vi "OG_1000_main__.vi"() -> ()   [LabVIEW 2015]
doc: "Программа мониторинга температуры ОГ-1000"
uses:
  <vilib>/NI/Modbus Library/API/Master/Modbus Master.lvclass
  <vilib>/Utility/error.llb/DialogType.ctl
panel:
  out "Связь с блоком 3":bool
  out "Связь с блоком 4":bool
  in  "Tab Control":enum32{"МНЕМОСХЕМА [K]", "R [Ом]", "НАСТРОЙКИ"}(tab)
  in  "dt 3_ch_visible":bool=TRUE
  in  "dt 2_ch_visible":bool=TRUE
  in  "dt 1_ch_visible":bool=TRUE
  out "dT3 2":dbl format="%.2f"
  out "dT2 2":dbl format="%.2f"
  out "dT1 2":dbl format="%.2f"
  in  "6_ch_visible":bool=TRUE
  in  "5_ch_visible":bool=TRUE
  in  "7_ch_visible":bool=TRUE
  in  "4_ch_visible":bool=TRUE
  in  "3_ch_visible":bool=TRUE
  in  "2_ch_visible":bool=TRUE
  in  "1_ch_visible":bool=TRUE
  out "T77":dbl format="%.2f"
  out "T66":dbl format="%.2f"
  out "T55":dbl format="%.2f"
  out "T44":dbl format="%.2f"
  out "T33":dbl format="%.2f"
  out "T22":dbl format="%.2f"
  out "T11":dbl format="%.2f"
  out "T7":dbl format="%.2f"
  out "dT3":dbl format="%.2f"
  out "T6":dbl format="%.2f"
  out "T5":dbl format="%.2f"
  out "dT2":dbl format="%.2f"
  out "T4":dbl format="%.2f"
  out "T3":dbl format="%.2f"
  out "T1":dbl format="%.2f"
  out "T2":dbl format="%.2f"
  out "dT1":dbl format="%.2f"
  out "R1":dbl format="%.2f"
  out "R2":dbl format="%.2f"
  out "R3":dbl format="%.2f"
  out "R6":dbl format="%.2f"
  out "R7":dbl format="%.2f"
  out "R5":dbl format="%.2f"
  out "R4":dbl format="%.2f"
  in  "Т min dt":dbl=4.0 min=-10.0 max=350.0 step=0.1
  in  "Т max dt":dbl=300.0 min=2.0 max=500.0 step=0.1
  in  "Autoscale dt":bool=TRUE
  in  "Порт Блока 3":u16
  in  "IP Блока 3":string
  out "Путь к файлу с коэф.":path
  in  "Пароль":string
  in  "настр. коэфф.":bool caption="Disconn"
  in  "Coeff_cl_ch5":T1 caption="T5" {"R0" format="%#_16g"; "k7" format="%#_16g"; "k6" format="%#_16g"; "k5" format="%#_16g"; "k4" format="%#_16g"; "k3" format="%#_16g"; "k2" format="%#_16g"; "k1" format="%#_16g"}
  in  "Coeff_cl_ch2":T1={"k1"=31.9101907935109921, "k2"=-399.867376562207937, "k3"=2119.32627579197288, "k4"=-5531.15447566658258, "k5"=7772.21873644739389, "k6"=-5292.23886113613844, "k7"=1613.2211984321475, "R0"=1613.2211984321475} caption="T2" {"R0" format="%#_16g"; "k7" format="%#_16g"; "k6" format="%#_16g"; "k5" format="%#_16g"; "k4" format="%#_16g"; "k3" format="%#_16g"; "k2" format="%#_16g"; "k1" format="%#_16g"}
  in  "load_coeff.":bool caption="Disconn"
  in  "save_coeff.":bool caption="Disconn"
  in  "Coeff_cl_ch4":T1 caption="T4" {"R0" format="%#_16g"; "k6" format="%#_16g"; "k5" format="%#_16g"; "k4" format="%#_16g"; "k3" format="%#_16g"; "k2" format="%#_16g"; "k1" format="%#_16g"; "k7" format="%#_16g"}
  in  "Coeff_cl_ch3":T1 caption="T3" {"R0" format="%#_16g"; "k6" format="%#_16g"; "k5" format="%#_16g"; "k4" format="%#_16g"; "k3" format="%#_16g"; "k2" format="%#_16g"; "k1" format="%#_16g"; "k7" format="%#_16g"}
  in  "Coeff_cl_ch6":T1 caption="T6" {"R0" format="%#_16g"; "k7" format="%#_16g"; "k6" format="%#_16g"; "k5" format="%#_16g"; "k4" format="%#_16g"; "k3" format="%#_16g"; "k2" format="%#_16g"; "k1" format="%#_16g"}
  in  "xScale -":bool
  in  "xScale +":bool
  out "мин.":string="1"
  in  "Добавить время":dbl(ring)=300.0 items=["10 сек."=10.0, "1 мин."=60.0, "5 мин."=300.0, "20 мин."=1200.0]
  out "часы":string="0"
  out "сек.":string="0"
  in  "stop":bool
  in  "Coeff_cl_ch1":T1 caption="T1" {"R0" format="%#_16g"; "k7" format="%#_16g"; "k6" format="%#_16g"; "k5" format="%#_16g"; "k4" format="%#_16g"; "k3" format="%#_16g"; "k2" format="%#_16g"; "k1" format="%#_16g"}
  in  "Coeff_cl_ch7":T1 caption="T7" {"R0" format="%#_16g"; "k7" format="%#_16g"; "k6" format="%#_16g"; "k5" format="%#_16g"; "k4" format="%#_16g"; "k3" format="%#_16g"; "k2" format="%#_16g"; "k1" format="%#_16g"}
  in  "GraphLookB":bool
  in  "Т min":dbl=4.0 min=-10.0 max=350.0 step=0.1
  in  "Т max":dbl=350.0 min=2.0 max=500.0 step=0.1
  in  "Autoscale":bool=TRUE
  in  "IP Блока 4":string
  in  "Порт Блока 4":u16
  out "Сутки":string
  in  "Запись в файл":bool
  out "Path":string
  out "File header exist?":bool caption="Disconn"
  in  "ADC_dyn_range":T2(ring)=enum."± 0.625 В"
  out "refnum out":refnum<file>
  out "Блок 3":refnum<class "Modbus Master.lvclass">
  out "Graphs T":dynamicdata(graph) caption="ИЗМЕРЕНИЯ ТЕМПЕРАТУРЫ, К"
  out "Блок 4":refnum<class "Modbus Master.lvclass">
  in  "Buf_size":u8=1 min=1 max=128
  in  "SPS":T3(ring)
  out "Graphs dT":dynamicdata(graph) caption="ПЕРЕПАДЫ ТЕМПЕРАТУР НА ТУРБОДЕТАНДЕРАХ, К"
  out "Расположение файла":path
  # "Блок 3"
  # "Блок 4"
  # "E51"
  # "X700"
  # "E52"
  # "D71"
  # "E53"
  # "D72"
  # "E54"
  # "X701"
  # "E61"
  # "X601"
  # "D60"
  # "C613"
  # "СБОРНИК"
  # "Шкала dТ"
  # ":"
  # ":"
  # "Шкала Т"
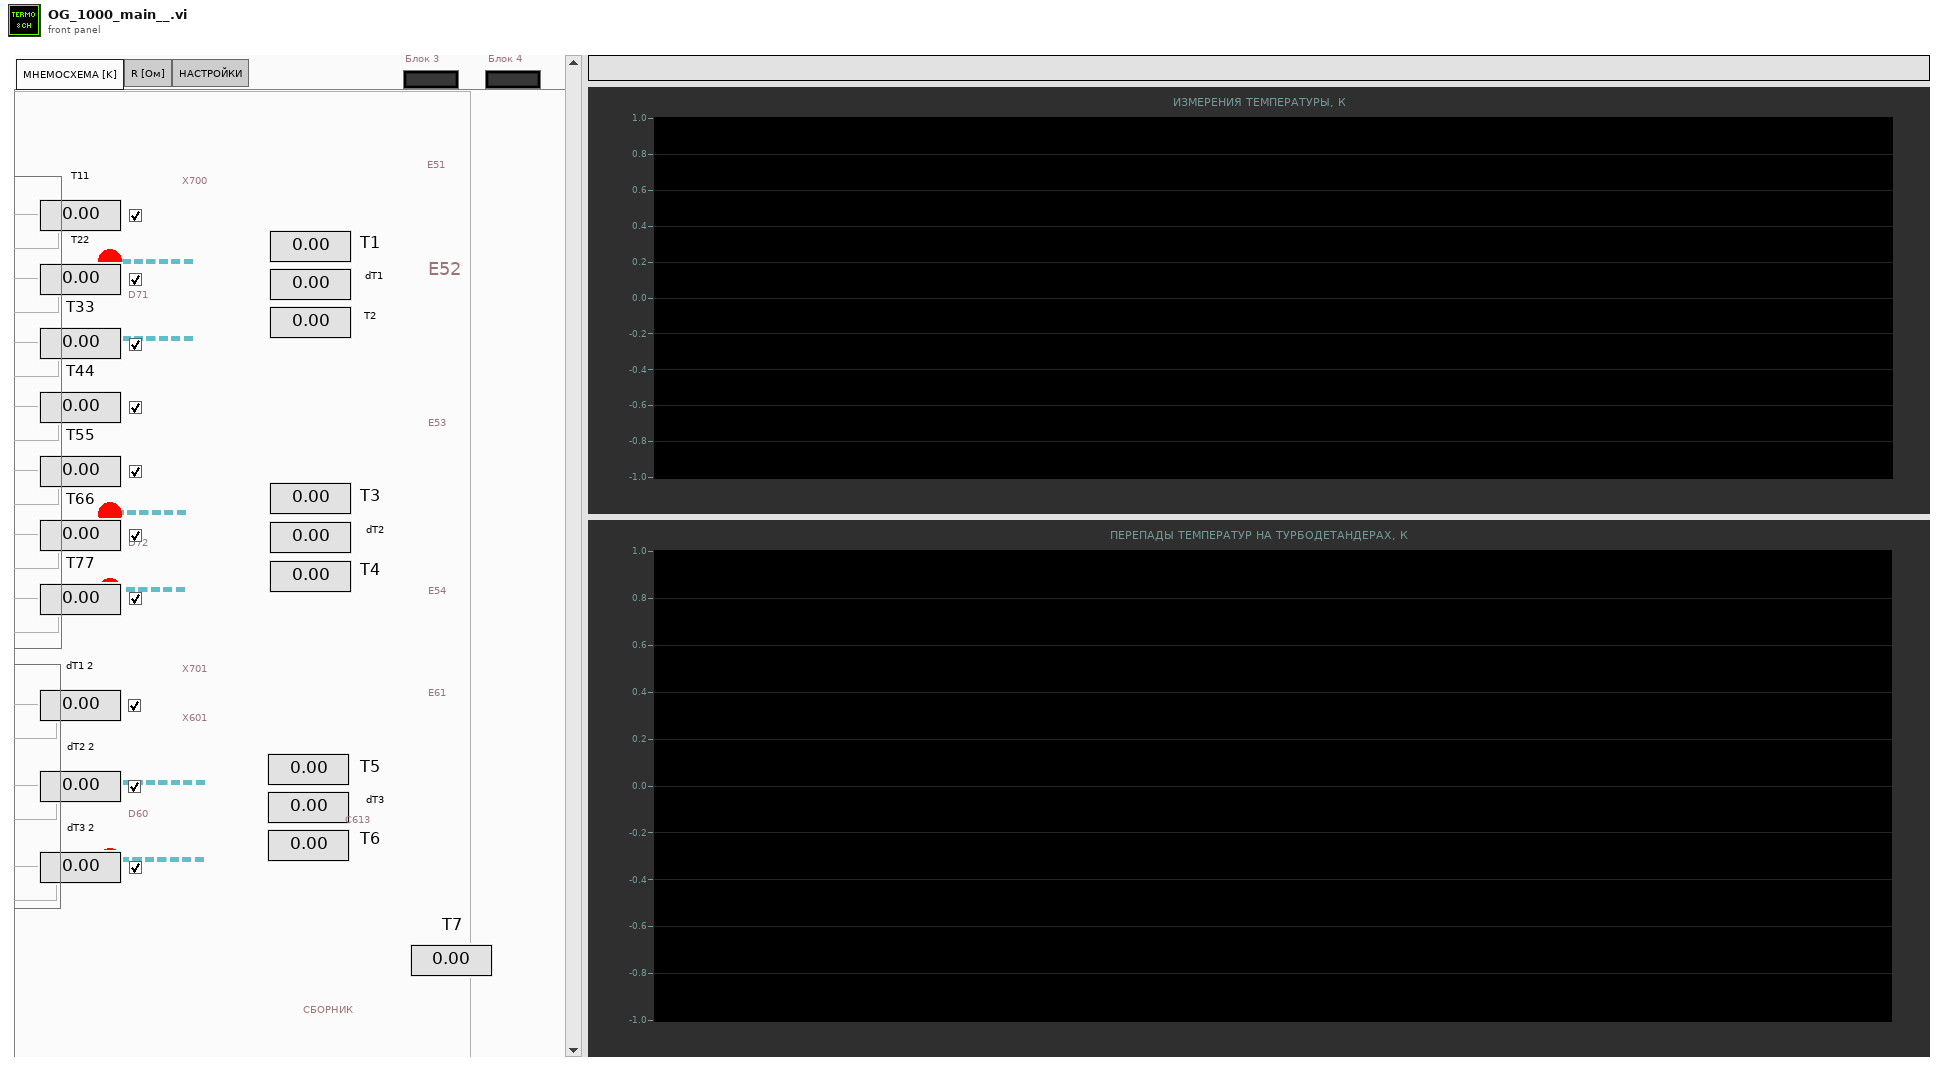
[diagram p1: front panel]
types:
  T1 = cluster{"k1":ext, "k2":ext, "k3":ext, "k4":ext, "k5":ext, "k6":ext, "k7":ext, "R0":ext}
  T2 = enum16{"± 5 В", "± 2.5 В", "± 1.25 В", "± 0.625 В", "± 312.5 мВ", "± 156.25 мВ", "± 78.125 мВ"}
  T3 = enum16{"2,5 SPS", "5 SPS", "10 SPS", "25 SPS", "50 SPS", "100 SPS", "500 SPS", "1 kSPS"}
  T4 = typedef "DialogType.ctl" = u16
  T5 = enum8{"Enabled", "Disabled", "Disabled and Grayed Out"}
  T6 = typedef "LVDateTimeRec.ctl" = cluster{"fractional second":dbl, "second":i32, "minute":i32, "hour":i32, "day of month":i32, "month":i32, "year":i32, "day of week":i32, "day of year":i32, "DST":i32}
  T7 = enum16{"open", "replace", "create", "open or create", "replace or create", "replace or create with confirmation"}
  T8 = cluster{"k1":ext, "k2":ext, "k3":ext, "k4":ext, "k5":ext, "k6":ext, "k7":ext, "R":ext}
  T9 = cluster{"T1":dbl, "T2":dbl, "T3":dbl, "T4":dbl, void, void}
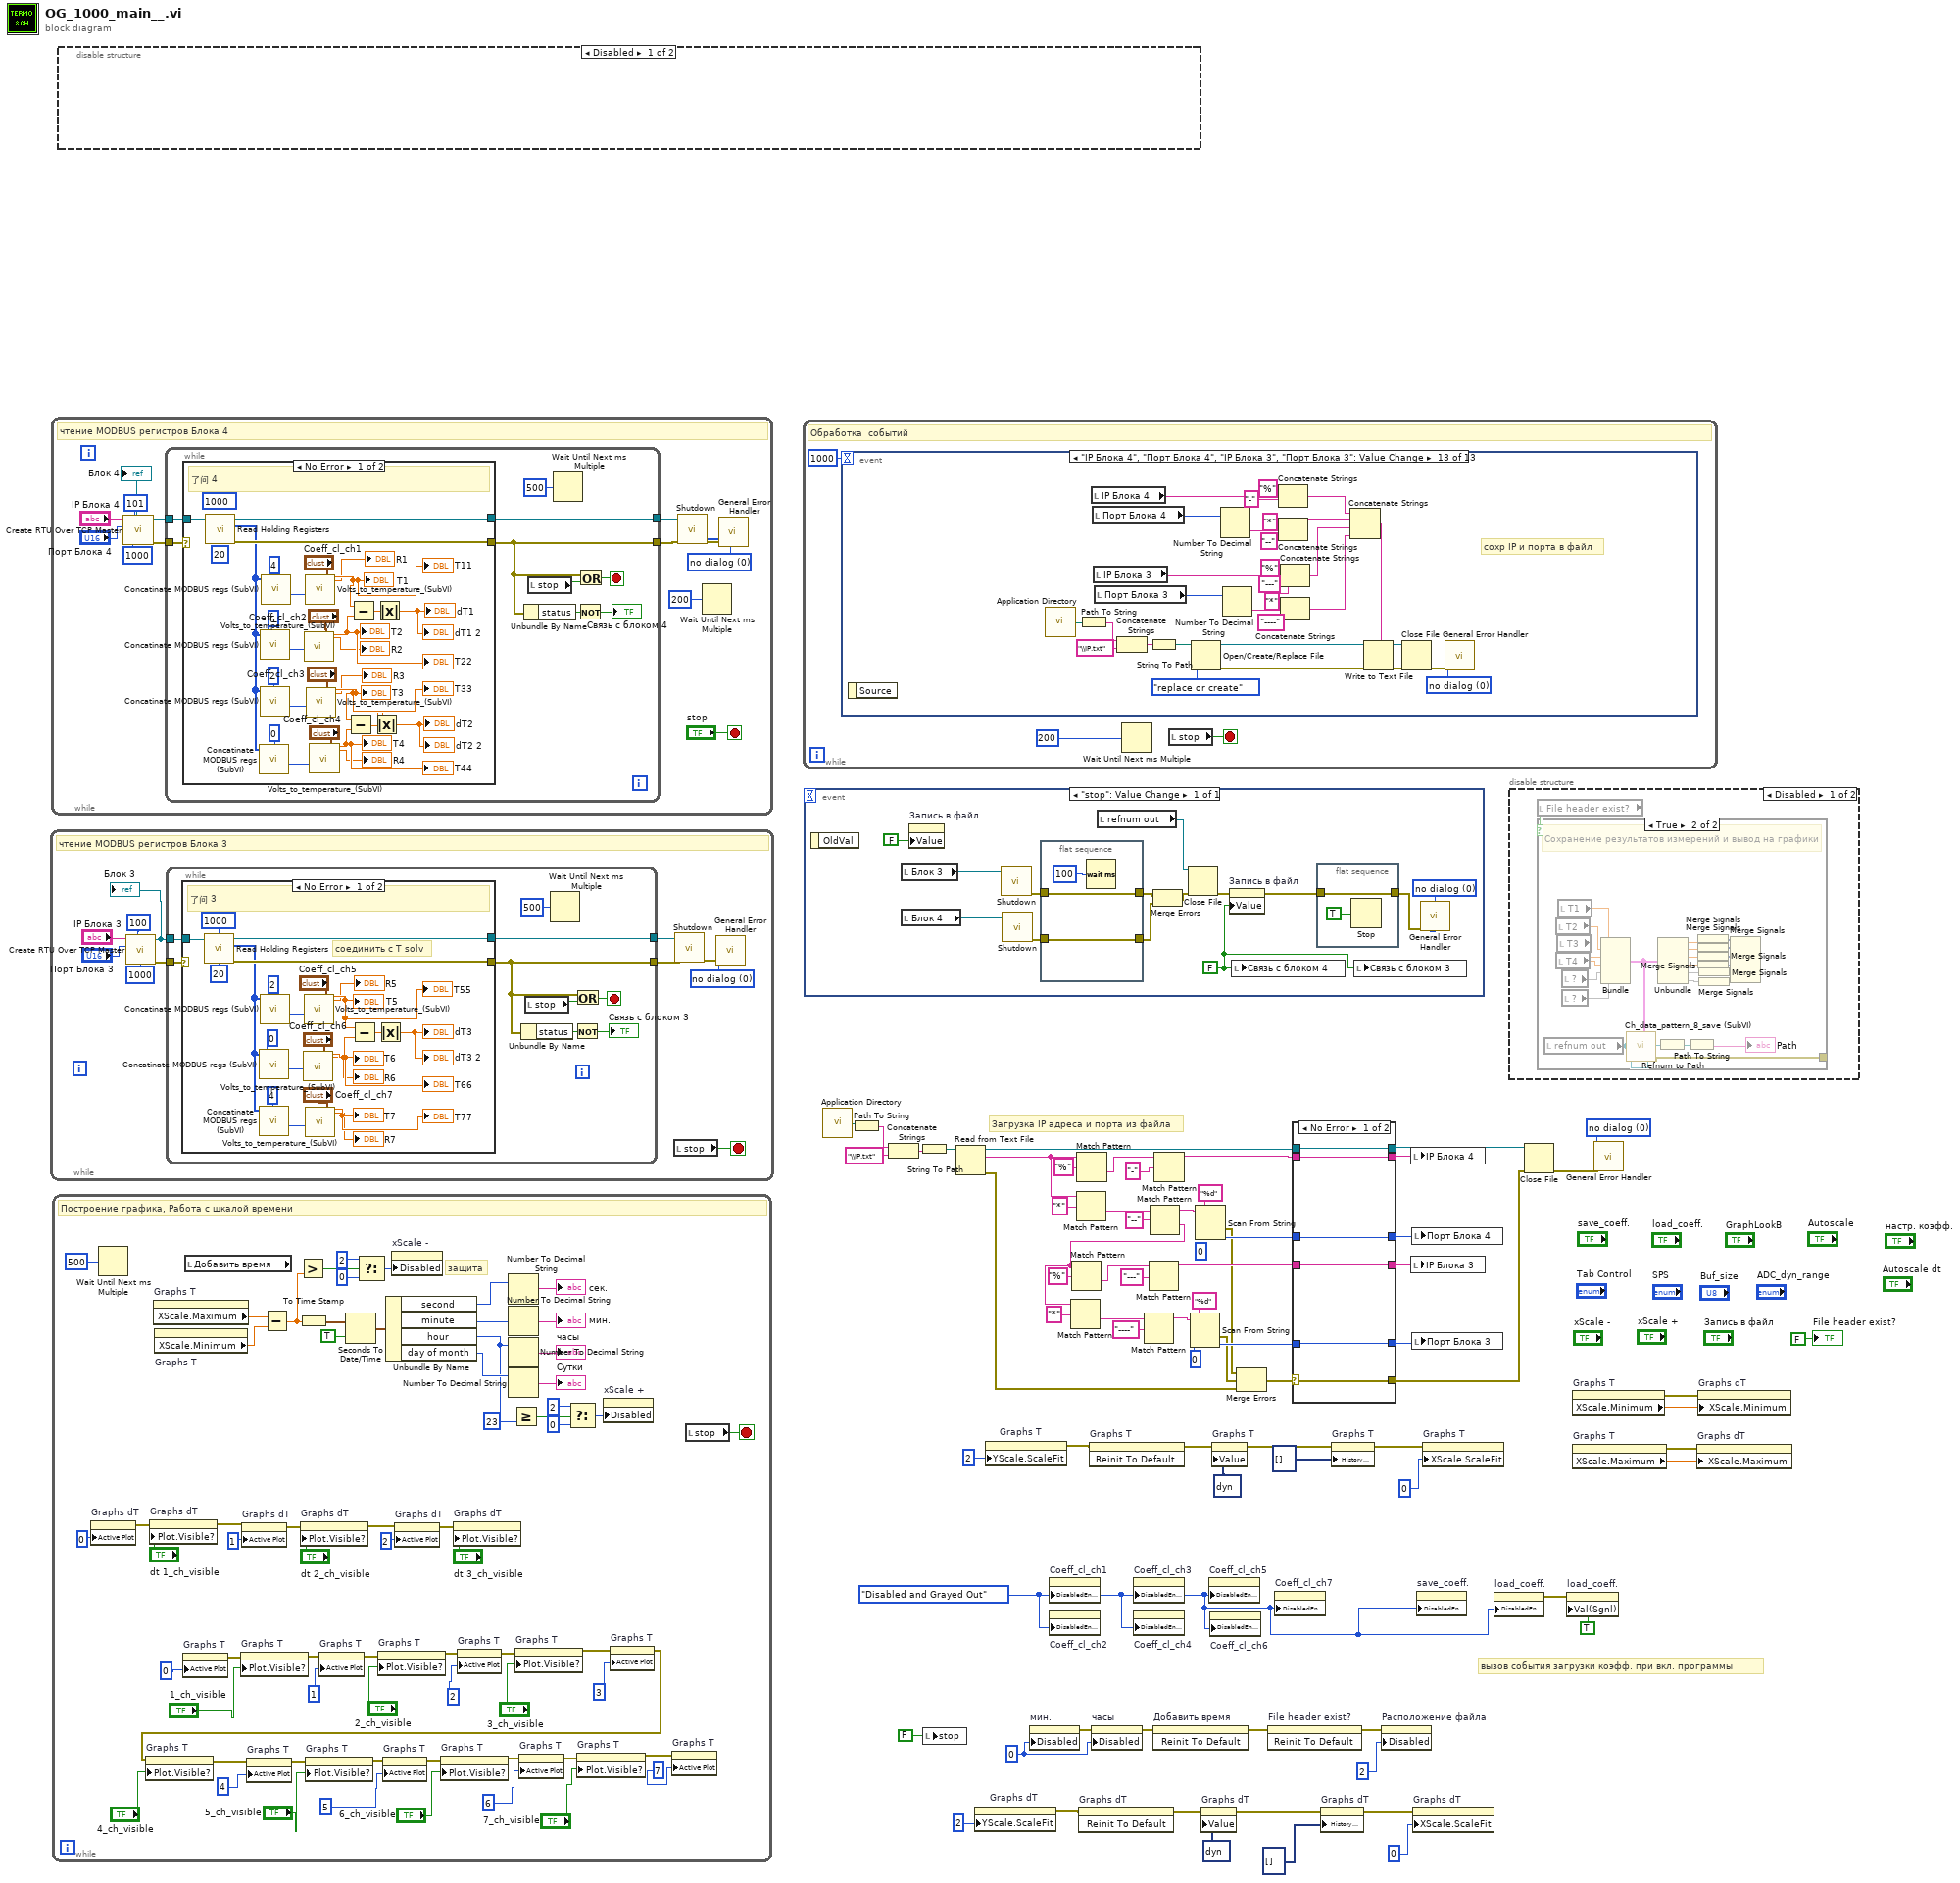
[diagram p0: block diagram]
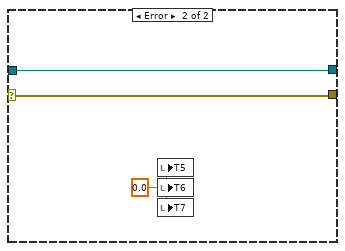
[diagram p2: hidden frame]
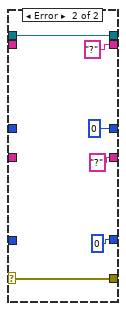
[diagram p3: hidden frame]
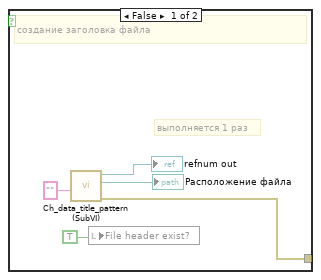
[diagram p5: hidden frame]
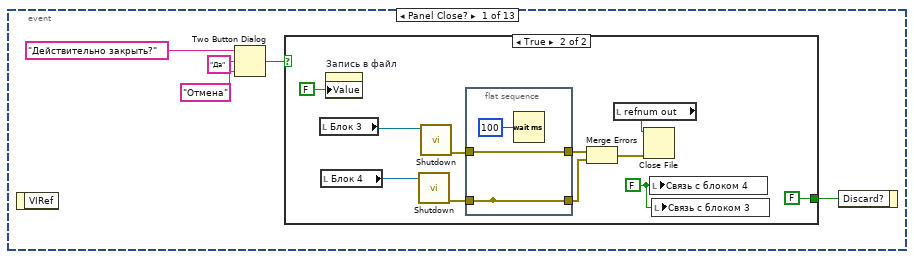
[diagram p7: hidden frame]
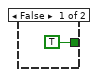
[diagram p8: hidden frame]
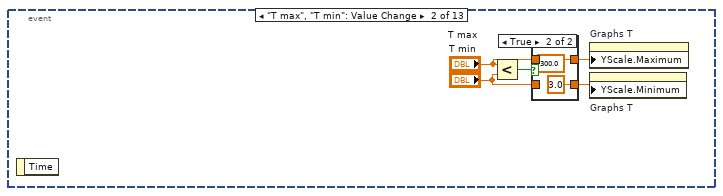
[diagram p9: hidden frame]
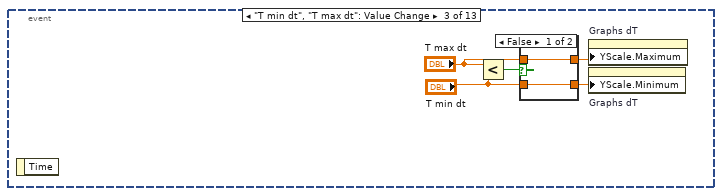
[diagram p11: hidden frame]
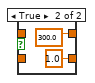
[diagram p12: hidden frame]
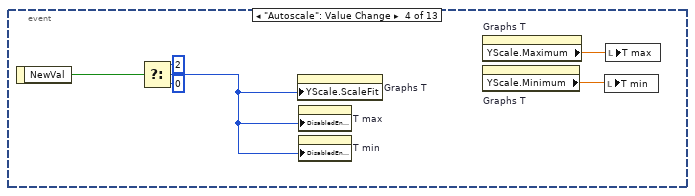
[diagram p13: hidden frame]
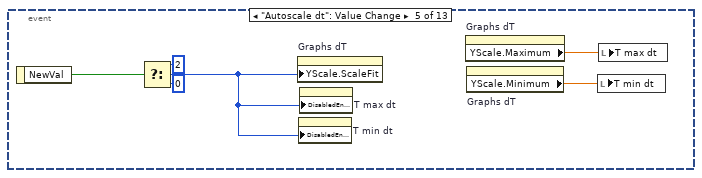
[diagram p14: hidden frame]
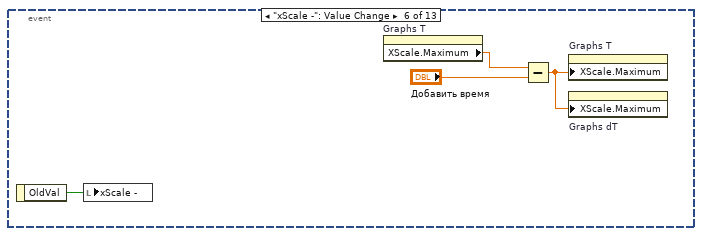
[diagram p15: hidden frame]
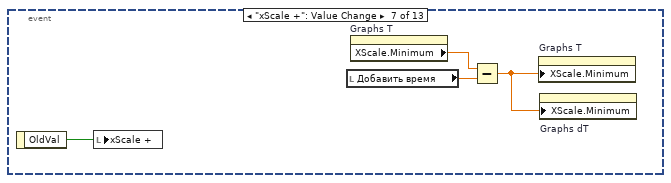
[diagram p16: hidden frame]
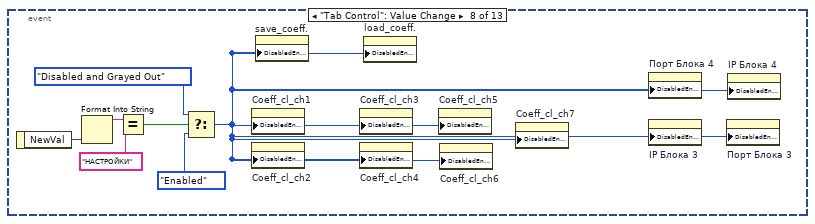
[diagram p17: hidden frame]
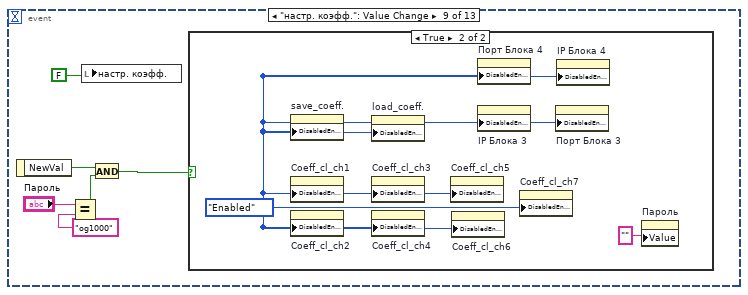
[diagram p18: hidden frame]
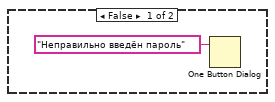
[diagram p19: hidden frame]
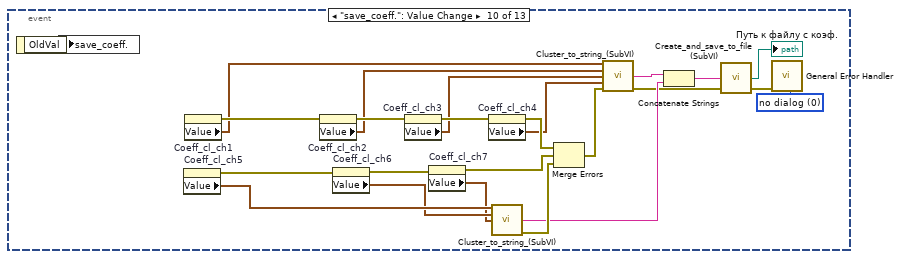
[diagram p20: hidden frame]
diagram:
  w14 = T4 0 items=["no dialog", "OK message", "continue or stop message", "OK message + warnings", "continue/stop + warnings"] ("type of dialog (OK msg:1)")
  w58 = T5."Disabled and Grayed Out" ("Disabled")
  w72 = u8 0 ("Disabled")
  # "Загрузка IP адреса и порта из файла"
  # "вызов события загрузки коэфф. при вкл. программы"
  n1 = while {
    stop <- w75 stop-if-true
    w76 = T4 0 items=["no dialog", "OK message", "continue or stop message", "OK message + warnings", "continue/stop + warnings"] ("type of dialog (OK msg:1)")
    # "чтение MODBUS регистров Блока 3"
    n2 = call "Create RTU Over TCP Master.vi"("unit ID"=u8 100 ("ID"), "connect timeout ms"=1000, "port (502)"="Порт Блока 3", "address"="IP Блока 3") -> ("error out"=w83:errorcluster, "TCP master instance"=w74:refnum<class "Modbus Master.lvclass">)  [unwired: 6 in]
    "Блок 3" <- w74
    n3 = while {
      tunnel: w74 -> [w93]
      tunnel: w83 -> [w92]
      tunnel: [w86] -> w79
      tunnel: [w91] -> w78
      stop <- w89 stop-if-true
      n4 = case shown="No Error" w92 {
        selector: w92 -> [_ w118]
        tunnel: w93 -> [w114 w119]
        tunnel: [w111 w118] -> w86
        tunnel: [w113 w119] -> w91
        frame No Error {
          # "соединить с T solv"
          # "了问 3"
          n5 = call-dynamic "Read Holding Registers.vi"("number of inputs"=u16 20, "starting address"=u16 1000, "Modbus master in"=w114) -> ("error out"=w111:errorcluster, "register values"=w107:u16[], "Modbus master out"=w113:refnum<class "Modbus Master.lvclass">)  [unwired: 6 in]
          n6 = call "Concatinate MODBUS regs (SubVI).vi"("LSB reg num"=u16 0, "registers array in"=w107) -> ("register data"=w108:i32)  [unwired: 8 in, 1 out]
          n7 = call "Concatinate MODBUS regs (SubVI).vi"("LSB reg num"=u16 4, "registers array in"=w107) -> ("register data"=w106:i32)  [unwired: 8 in, 1 out]
          n8 = call "Concatinate MODBUS regs (SubVI).vi"("LSB reg num"=u16 2, "registers array in"=w107) -> ("register data"=w110:i32)  [unwired: 8 in, 1 out]
          n9 = call "Volts_to_temperature_(SubVI).vi"("Resistance"=w108, "koeff. cluster"="Coeff_cl_ch6") -> ("T solvation"=w98:dbl, "meas_voltage"=→"R6":dbl)  [unwired: 21 in, 3 out]
          "T6" <- w98
          "T66" <- w98
          n10 = call "Volts_to_temperature_(SubVI).vi"("Resistance"=w110, "koeff. cluster"="Coeff_cl_ch5") -> ("T solvation"=w99:dbl, "meas_voltage"=→"R5":dbl)  [unwired: 21 in, 3 out]
          "T5" <- w99
          "T55" <- w99
          n11 = call "Volts_to_temperature_(SubVI).vi"("Resistance"=w106, "koeff. cluster"="Coeff_cl_ch7") -> ("T solvation"=→"T7" →"T77":dbl, "meas_voltage"=→"R7":dbl)  [unwired: 21 in, 3 out]
          n12 = Subtract(x=w99, y=w98) -> (x-y=w101:dbl)
          n13 = Absolute Value(x=w101) -> (abs(x)=→"dT3" →"dT3 2":dbl)
        }
        frame Error {
          w117 = 0.0 ("T6")
          n14 = local write "T5"(w117) -> ()
          n15 = local write "T6"(w117) -> ()
          n16 = local write "T7"(w117) -> ()
        }
      }
      n17 = Unbundle By Name(w86) -> ("status"=w88:bool)
      n18 = local read "stop"() -> (w90:bool)
      n19 = Wait Until Next ms Multiple(millisecond multiple=u32 500) -> ()  [unwired: 1 out]
      n20 = Not(x=w88) -> (.not. x?=→"Связь с блоком 3":bool)
      n21 = Or(x=w86, y=w90) -> (x .or. y?=w89:bool)
    }
    n22 = local read "stop"() -> (w75:bool)
    n23 = call-dynamic "Shutdown.vi"("error in"=w79, "Modbus master in"=w78) -> ("error out"=w80:errorcluster)  [unwired: 9 in]
    n24 = call <vilib>:"General Error Handler.vi"("type of dialog (OK msg:1)"=w76, "error in (no error)"=w80) -> ()  [unwired: 1 in, 13 out]
  }
  n25 = while {
    stop <- "stop" stop-if-true
    w120 = T4 0 items=["no dialog", "OK message", "continue or stop message", "OK message + warnings", "continue/stop + warnings"] ("type of dialog (OK msg:1)")
    # "чтение MODBUS регистров Блока 4"
    n26 = call "Create RTU Over TCP Master.vi"("unit ID"=u8 101 ("ID"), "connect timeout ms"=1000, "port (502)"="Порт Блока 4", "address"="IP Блока 4") -> ("error out"=w124:errorcluster, "TCP master instance"=w125:refnum<class "Modbus Master.lvclass">)  [unwired: 6 in]
    "Блок 4" <- w125
    n27 = while {
      tunnel: w125 -> [w140]
      tunnel: w124 -> [w139]
      tunnel: [w133] -> w123
      tunnel: [w138] -> w122
      stop <- w136 stop-if-true
      n28 = case shown="No Error" w139 {
        selector: w139 -> [_ w172]
        tunnel: w140 -> [w168 w173]
        tunnel: [w165 w172] -> w133
        tunnel: [w167 w173] -> w138
        frame No Error {
          # "了问 4"
          n29 = call-dynamic "Read Holding Registers.vi"("number of inputs"=u16 20, "starting address"=u16 1000, "Modbus master in"=w168) -> ("error out"=w165:errorcluster, "register values"=w159:u16[], "Modbus master out"=w167:refnum<class "Modbus Master.lvclass">)  [unwired: 6 in]
          n30 = call "Concatinate MODBUS regs (SubVI).vi"("LSB reg num"=u16 0, "registers array in"=w159) -> ("register data"=w154:i32)  [unwired: 8 in, 1 out]
          n31 = call "Concatinate MODBUS regs (SubVI).vi"("LSB reg num"=u16 6, "registers array in"=w159) -> ("register data"=w161:i32)  [unwired: 8 in, 1 out]
          n32 = call "Concatinate MODBUS regs (SubVI).vi"("LSB reg num"=u16 2, "registers array in"=w159) -> ("register data"=w156:i32)  [unwired: 8 in, 1 out]
          n33 = call "Concatinate MODBUS regs (SubVI).vi"("LSB reg num"=u16 4, "registers array in"=w159) -> ("register data"=w163:i32)  [unwired: 8 in, 1 out]
          n34 = call "Volts_to_temperature_(SubVI).vi"("Resistance"=w161, "koeff. cluster"="Coeff_cl_ch2") -> ("T solvation"=w148:dbl, "meas_voltage"=→"R2":dbl)  [unwired: 21 in, 3 out]
          "T2" <- w148
          "T22" <- w148
          n35 = call "Volts_to_temperature_(SubVI).vi"("Resistance"=w163, "koeff. cluster"="Coeff_cl_ch1") -> ("T solvation"=w149:dbl, "meas_voltage"=→"R1":dbl)  [unwired: 21 in, 3 out]
          "T1" <- w149
          "T11" <- w149
          n36 = call "Volts_to_temperature_(SubVI).vi"("Resistance"=w156, "koeff. cluster"="Coeff_cl_ch3") -> ("T solvation"=w147:dbl, "meas_voltage"=→"R3":dbl)  [unwired: 21 in, 3 out]
          "T3" <- w147
          "T33" <- w147
          n37 = call "Volts_to_temperature_(SubVI).vi"("Resistance"=w154, "koeff. cluster"="Coeff_cl_ch4") -> ("T solvation"=w146:dbl, "meas_voltage"=→"R4":dbl)  [unwired: 21 in, 3 out]
          "T4" <- w146
          "T44" <- w146
          n38 = Subtract(x=w147, y=w146) -> (x-y=w142:dbl)
          n39 = Subtract(x=w149, y=w148) -> (x-y=w152:dbl)
          n40 = Absolute Value(x=w142) -> (abs(x)=→"dT2" →"dT2 2":dbl)
          n41 = Absolute Value(x=w152) -> (abs(x)=→"dT1" →"dT1 2":dbl)
        }
        frame Error {
          w171 = 0.0 ("T1")
          n42 = local write "T1"(w171) -> ()
          n43 = local write "T2"(w171) -> ()
          n44 = local write "T3"(w171) -> ()
          n45 = local write "T4"(w171) -> ()
        }
      }
      n46 = Unbundle By Name(w133) -> ("status"=w135:bool)
      n47 = local read "stop"() -> (w137:bool)
      n48 = Wait Until Next ms Multiple(millisecond multiple=u32 500) -> ()  [unwired: 1 out]
      n49 = Not(x=w135) -> (.not. x?=→"Связь с блоком 4":bool)
      n50 = Or(x=w133, y=w137) -> (x .or. y?=w136:bool)
    }
    n51 = call-dynamic "Shutdown.vi"("error in"=w123, "Modbus master in"=w122) -> ("error out"=w121:errorcluster)  [unwired: 9 in]
    n52 = Wait Until Next ms Multiple(millisecond multiple=u32 200) -> ()  [unwired: 1 out]
    n53 = call <vilib>:"General Error Handler.vi"("type of dialog (OK msg:1)"=w120, "error in (no error)"=w121) -> ()  [unwired: 1 in, 13 out]
  }
  n54 = while {
    stop <- w239 stop-if-true
    # "защита"
    # "Построение графика, Работа с шкалой времени"
    n55 = property on="Graphs dT" class="WFChart (strict)"("Active Plot"=u32 0) -> (error out=w184:errorcluster)  [unwired: 2 in, 1 out]
    n56 = Wait Until Next ms Multiple(millisecond multiple=u32 500) -> ()  [unwired: 1 out]
    n57 = property on="Graphs dT" class="WFChart (strict)"(error in=w184, "Plot.Visible?"="dt 1_ch_visible") -> (error out=w178:errorcluster)  [unwired: 1 in, 1 out]
    n58 = property on="Graphs T" class="WFChart (strict)"() -> ("XScale.Maximum"=w215:dbl)  [unwired: 2 in, 2 out]
    n59 = property on="Graphs T" class="WFChart (strict)"() -> ("XScale.Minimum"=w214:dbl)  [unwired: 2 in, 2 out]
    n60 = property on="Graphs T" class="WFChart (strict)"("Active Plot"=u32 0) -> (error out=w187:errorcluster)  [unwired: 2 in, 1 out]
    n61 = local read "Добавить время"() -> (w238:dbl)
    n62 = property on="Graphs T" class="WFChart (strict)"(error in=w187, "Plot.Visible?"="1_ch_visible") -> (error out=w193:errorcluster)  [unwired: 1 in, 1 out]
    n63 = property on="Graphs dT" class="WFChart (strict)"(error in=w178, "Active Plot"=u32 1) -> (error out=w179:errorcluster)  [unwired: 1 in, 1 out]
    n64 = Subtract(x=w215, y=w214) -> (x-y=w228:dbl)
    n65 = Greater?(x=w238, y=w228) -> (0:w221:bool)
    n66 = To Time Stamp(1:w228) -> (0:w236:timestamp)
    n67 = property on="Graphs dT" class="WFChart (strict)"(error in=w179, "Plot.Visible?"="dt 2_ch_visible") -> (error out=w174:errorcluster)  [unwired: 1 in, 1 out]
    n68 = property on="Graphs T" class="WFChart (strict)"(error in=w193, "Active Plot"=u32 1) -> (error out=w190:errorcluster)  [unwired: 1 in, 1 out]
    n69 = Seconds To Date/Time(time stamp (now)=w236, to UTC (F)=TRUE) -> (date time rec=w235:T6)
    n70 = Select(t=u8 2 ("Disabled"), s=w221, f=u8 0 ("Disabled")) -> (s? t:f=w224:u8)
    n71 = property on="Graphs T" class="WFChart (strict)"(error in=w190, "Plot.Visible?"="2_ch_visible") -> (error out=w196:errorcluster)  [unwired: 1 in, 1 out]
    n72 = Unbundle By Name(w235) -> ("second"=w234:i32, "minute"=w233:i32, "hour"=w226:i32, "day of month"=w232:i32)
    n73 = property on="xScale -" class="Bool (strict)"("Disabled"=w224) -> ()  [unwired: 2 in, 2 out]
    n74 = property on="Graphs dT" class="WFChart (strict)"(error in=w174, "Active Plot"=u32 2) -> (error out=w177:errorcluster)  [unwired: 1 in, 1 out]
    n75 = property on="Graphs dT" class="WFChart (strict)"(error in=w177, "Plot.Visible?"="dt 3_ch_visible") -> ()  [unwired: 1 in, 2 out]
    n76 = property on="Graphs T" class="WFChart (strict)"(error in=w196, "Active Plot"=u32 2) -> (error out=w191:errorcluster)  [unwired: 1 in, 1 out]
    n77 = Number To Decimal String(number=w234) -> (decimal integer string=→"сек.":string)  [unwired: 1 out]
    n78 = Number To Decimal String(number=w233) -> (decimal integer string=→"мин.":string)  [unwired: 1 out]
    n79 = Number To Decimal String(number=w226) -> (decimal integer string=→"часы":string)  [unwired: 1 out]
    n80 = Number To Decimal String(number=w232) -> (decimal integer string=→"Сутки":string)  [unwired: 1 out]
    n81 = Greater Or Equal?(x=w226, y=23) -> (x >= y?=w217:bool)
    n82 = property on="Graphs T" class="WFChart (strict)"(error in=w191, "Plot.Visible?"="3_ch_visible") -> (error out=w199:errorcluster)  [unwired: 1 in, 1 out]
    n83 = Select(t=u8 2 ("Disabled"), s=w217, f=u8 0 ("Disabled")) -> (s? t:f=w220:u8)
    n84 = property on="xScale +" class="Bool (strict)"("Disabled"=w220) -> ()  [unwired: 2 in, 2 out]
    n85 = property on="Graphs T" class="WFChart (strict)"(error in=w199, "Active Plot"=u32 3) -> (error out=w185:errorcluster)  [unwired: 1 in, 1 out]
    n86 = property on="Graphs T" class="WFChart (strict)"(error in=w185, "Plot.Visible?"="4_ch_visible") -> (error out=w208:errorcluster)  [unwired: 1 in, 1 out]
    n87 = property on="Graphs T" class="WFChart (strict)"(error in=w208, "Active Plot"=u32 4) -> (error out=w206:errorcluster)  [unwired: 1 in, 1 out]
    n88 = property on="Graphs T" class="WFChart (strict)"(error in=w206, "Plot.Visible?"="5_ch_visible") -> (error out=w203:errorcluster)  [unwired: 1 in, 1 out]
    n89 = property on="Graphs T" class="WFChart (strict)"(error in=w203, "Active Plot"=u32 5) -> (error out=w205:errorcluster)  [unwired: 1 in, 1 out]
    n90 = property on="Graphs T" class="WFChart (strict)"(error in=w205, "Plot.Visible?"="6_ch_visible") -> (error out=w202:errorcluster)  [unwired: 1 in, 1 out]
    n91 = property on="Graphs T" class="WFChart (strict)"(error in=w202, "Active Plot"=u32 6) -> (error out=w204:errorcluster)  [unwired: 1 in, 1 out]
    n92 = property on="Graphs T" class="WFChart (strict)"(error in=w204, "Plot.Visible?"="7_ch_visible") -> (error out=w201:errorcluster)  [unwired: 1 in, 1 out]
    n93 = property on="Graphs T" class="WFChart (strict)"(error in=w201, "Active Plot"=u32 7) -> ()  [unwired: 1 in, 2 out]
    n94 = local read "stop"() -> (w239:bool)
  }
  n95 = disable-structure shown="Disabled" {
    frame Disabled {
    }
    frame Enabled {
    }
  }
  n96 = while {
    stop <- w241 stop-if-true
    # "Обработка  событий"
    n97 = event shown="[12] \"IP Блока 4\", \"Порт Блока 4\", \"IP Блока 3\", \"Порт Блока 3\": Value Change" {
      selector: _ -> [_ _ _ _ _ _ _ _ _ _ _ _ _]
      dyn-events: _ -> [_ _ _ _ _ _ _ _ _ _ _ _ _]
      timeout: 1000 -> [_ _ _ _ _ _ _ _ _ _ _ _ _]
      event Panel Close? {
        n98 = event-data() -> ()  [unwired: 2 out]
        n99 = Two Button Dialog(message="Действительно закрыть?", 1:"Отмена" ("T button name (\"OK\")"), 2:"Да" ("T button name (\"OK\")")) -> (T button?=w247:bool)
        n100 = case shown="True" w247 {
          tunnel: [TRUE ("Discard?") FALSE ("Discard?")] -> w243
          frame False {
          }
          frame True {
            w249 = FALSE ("Связь с блоком 4")
            n101 = local read "Блок 3"() -> (w255:refnum<class "Modbus Master.lvclass">)
            n102 = local read "Блок 4"() -> (w254:refnum<class "Modbus Master.lvclass">)
            n103 = property on="Запись в файл" class="Bool (strict)"("Value"=FALSE ("Запись в файл")) -> ()  [unwired: 2 in, 2 out]
            n104 = call-dynamic "Shutdown.vi"("Modbus master in"=w254) -> ("error out"=w253:errorcluster)  [unwired: 10 in]
            n105 = call-dynamic "Shutdown.vi"("Modbus master in"=w255) -> ("error out"=w256:errorcluster)  [unwired: 10 in]
            n106 = flat-sequence {
              tunnel: [w261] -> w252
              tunnel: w256 -> [w261]
              tunnel: w253 -> [w260]
              tunnel: [w260] -> _
              tunnel: [w260] -> w251
              frame #0 {
                n107 = Wait (ms)(milliseconds to wait=u32 100) -> ()  [unwired: 1 out]
              }
            }
            n108 = Merge Errors(w252, w251) -> (w250:errorcluster)
            n109 = local read "refnum out"() -> (w258:refnum<file>)
            n110 = Close File(refnum=w258, error in=w250) -> ()  [unwired: 2 out]
            n111 = local write "Связь с блоком 4"(w249) -> ()
            n112 = local write "Связь с блоком 3"(w249) -> ()
          }
        }
        n113 = event-data("Discard?"=w243) -> ()  [unwired: 1 in, 1 out]
      }
      event "Т max", "Т min": Value Change {
        n114 = event-data() -> ()  [unwired: 2 out]
        n115 = Less?(x="Т max", y="Т min") -> (x < y?=w267:bool)
        n116 = case shown="True" w267 {
          tunnel: [w268 300.0 ("x+1")] -> w265
          tunnel: [w269 3.0 ("x+1")] -> w266
          tunnel: "Т max" -> [w268 _]
          tunnel: "Т min" -> [w269 _]
          frame False {
          }
          frame True {
          }
        }
        n117 = property on="Graphs T" class="WFChart (strict)"("YScale.Maximum"=w265) -> ()  [unwired: 2 in, 2 out]
        n118 = property on="Graphs T" class="WFChart (strict)"("YScale.Minimum"=w266) -> ()  [unwired: 2 in, 2 out]
      }
      event "Т min dt", "Т max dt": Value Change {
        n119 = event-data() -> ()  [unwired: 2 out]
        n120 = Less?(x="Т max dt", y="Т min dt") -> (x < y?=w276:bool)
        n121 = case shown="False" w276 {
          tunnel: [w277 300.0 ("x+1")] -> w273
          tunnel: [w278 1.0 ("x+1")] -> w272
          tunnel: "Т max dt" -> [w277 _]
          tunnel: "Т min dt" -> [w278 _]
          frame False {
          }
          frame True {
          }
        }
        n122 = property on="Graphs dT" class="WFChart (strict)"("YScale.Maximum"=w273) -> ()  [unwired: 2 in, 2 out]
        n123 = property on="Graphs dT" class="WFChart (strict)"("YScale.Minimum"=w272) -> ()  [unwired: 2 in, 2 out]
      }
      event "Autoscale": Value Change {
        n124 = event-data() -> ("NewVal"=w281:bool)  [unwired: 1 out]
        n125 = Select(t=u8 2 ("Y Scale.Scale Fit"), s=w281, f=u8 0 ("Y Scale.Scale Fit")) -> (s? t:f=w284:u8)
        n126 = property on="Graphs T" class="WFChart (strict)"("YScale.ScaleFit"=w284) -> ()  [unwired: 2 in, 2 out]
        n127 = property on="Т max" class="DigNum (strict)"("DisabledEnum"=w284) -> ()  [unwired: 2 in, 2 out]
        n128 = property on="Т min" class="DigNum (strict)"("DisabledEnum"=w284) -> ()  [unwired: 2 in, 2 out]
        n129 = property on="Graphs T" class="WFChart (strict)"() -> ("YScale.Maximum"=w286:dbl)  [unwired: 2 in, 2 out]
        n130 = property on="Graphs T" class="WFChart (strict)"() -> ("YScale.Minimum"=w285:dbl)  [unwired: 2 in, 2 out]
        n131 = local write "Т min"(w285) -> ()
        n132 = local write "Т max"(w286) -> ()
      }
      event "Autoscale dt": Value Change {
        n133 = event-data() -> ("NewVal"=w290:bool)  [unwired: 1 out]
        n134 = Select(t=u8 2 ("Y Scale.Scale Fit"), s=w290, f=u8 0 ("Y Scale.Scale Fit")) -> (s? t:f=w287:u8)
        n135 = property on="Graphs dT" class="WFChart (strict)"("YScale.ScaleFit"=w287) -> ()  [unwired: 2 in, 2 out]
        n136 = property on="Т min dt" class="DigNum (strict)"("DisabledEnum"=w287) -> ()  [unwired: 2 in, 2 out]
        n137 = property on="Т max dt" class="DigNum (strict)"("DisabledEnum"=w287) -> ()  [unwired: 2 in, 2 out]
        n138 = property on="Graphs dT" class="WFChart (strict)"() -> ("YScale.Maximum"=w289:dbl)  [unwired: 2 in, 2 out]
        n139 = property on="Graphs dT" class="WFChart (strict)"() -> ("YScale.Minimum"=w288:dbl)  [unwired: 2 in, 2 out]
        n140 = local write "Т min dt"(w288) -> ()
        n141 = local write "Т max dt"(w289) -> ()
      }
      event "xScale -": Value Change {
        n142 = event-data() -> ("OldVal"=w296:bool)  [unwired: 1 out]
        n143 = local write "xScale -"(w296) -> ()
        n144 = property on="Graphs T" class="WFChart (strict)"() -> ("XScale.Maximum"=w294:dbl)  [unwired: 2 in, 2 out]
        n145 = Subtract(x=w294, y="Добавить время") -> (x-y=w293:dbl)
        n146 = property on="Graphs T" class="WFChart (strict)"("XScale.Maximum"=w293) -> ()  [unwired: 2 in, 2 out]
        n147 = property on="Graphs dT" class="WFChart (strict)"("XScale.Maximum"=w293) -> ()  [unwired: 2 in, 2 out]
      }
      event "xScale +": Value Change {
        n148 = event-data() -> ("OldVal"=w300:bool)  [unwired: 1 out]
        n149 = local write "xScale +"(w300) -> ()
        n150 = local read "Добавить время"() -> (w299:dbl)
        n151 = property on="Graphs T" class="WFChart (strict)"() -> ("XScale.Minimum"=w298:dbl)  [unwired: 2 in, 2 out]
        n152 = Subtract(x=w298, y=w299) -> (x-y=w297:dbl)
        n153 = property on="Graphs T" class="WFChart (strict)"("XScale.Minimum"=w297) -> ()  [unwired: 2 in, 2 out]
        n154 = property on="Graphs dT" class="WFChart (strict)"("XScale.Minimum"=w297) -> ()  [unwired: 2 in, 2 out]
      }
      event "Tab Control": Value Change {
        n155 = event-data() -> ("NewVal"=w307:enum32{"МНЕМОСХЕМА [K]", "R [Ом]", "НАСТРОЙКИ"})  [unwired: 1 out]
        n156 = Format Into String(w307) -> (resulting string=w306:string)  [unwired: 3 in, 1 out]
        n157 = Equal?(x=w306, y="НАСТРОЙКИ") -> (x = y?=w304:bool)
        n158 = Select(t=T5."Disabled and Grayed Out" ("Disabled"), s=w304, f=T5."Enabled" ("Disabled")) -> (s? t:f=w301:T5)
        n159 = property on="Coeff_cl_ch1" class="Clust (strict)"("DisabledEnum"=w301) -> ()  [unwired: 2 in, 2 out]
        n160 = property on="Coeff_cl_ch2" class="Clust (strict)"("DisabledEnum"=w301) -> ()  [unwired: 2 in, 2 out]
        n161 = property on="save_coeff." class="Bool (strict)"("DisabledEnum"=w301) -> ()  [unwired: 2 in, 2 out]
        n162 = property on="Coeff_cl_ch3" class="Clust (strict)"("DisabledEnum"=w301) -> ()  [unwired: 2 in, 2 out]
        n163 = property on="Coeff_cl_ch4" class="Clust (strict)"("DisabledEnum"=w301) -> ()  [unwired: 2 in, 2 out]
        n164 = property on="load_coeff." class="Bool (strict)"("DisabledEnum"=w301) -> ()  [unwired: 2 in, 2 out]
        n165 = property on="Coeff_cl_ch5" class="Clust (strict)"("DisabledEnum"=w301) -> ()  [unwired: 2 in, 2 out]
        n166 = property on="Coeff_cl_ch6" class="Clust (strict)"("DisabledEnum"=w301) -> ()  [unwired: 2 in, 2 out]
        n167 = property on="Coeff_cl_ch7" class="Clust (strict)"("DisabledEnum"=w301) -> ()  [unwired: 2 in, 2 out]
        n168 = property on="Порт Блока 4" class="DigNum (strict)"("DisabledEnum"=w301) -> ()  [unwired: 2 in, 2 out]
        n169 = property on="IP Блока 3" class="Str"("DisabledEnum"=w301) -> ()  [unwired: 2 in, 2 out]
        n170 = property on="Порт Блока 3" class="DigNum (strict)"("DisabledEnum"=w301) -> ()  [unwired: 2 in, 2 out]
        n171 = property on="IP Блока 4" class="Str"("DisabledEnum"=w301) -> ()  [unwired: 2 in, 2 out]
      }
      event "настр. коэфф.": Value Change {
        n172 = event-data() -> ("NewVal"=w313:bool)  [unwired: 1 out]
        n173 = Equal?(x="Пароль", y="og1000") -> (x = y?=w310:bool)
        n174 = local write "настр. коэфф."(FALSE ("насстр. коэфф.")) -> ()
        n175 = And(x=w313, y=w310) -> (x .and. y?=w309:bool)
        n176 = case shown="True" w309 {
          frame False {
            n177 = One Button Dialog(message="Неправильно введён пароль") -> ()  [unwired: 1 in, 1 out]
          }
          frame True {
            w315 = T5."Enabled" ("Disabled")
            n178 = property on="save_coeff." class="Bool (strict)"("DisabledEnum"=w315) -> ()  [unwired: 2 in, 2 out]
            n179 = property on="Coeff_cl_ch1" class="Clust (strict)"("DisabledEnum"=w315) -> ()  [unwired: 2 in, 2 out]
            n180 = property on="Coeff_cl_ch2" class="Clust (strict)"("DisabledEnum"=w315) -> ()  [unwired: 2 in, 2 out]
            n181 = property on="load_coeff." class="Bool (strict)"("DisabledEnum"=w315) -> ()  [unwired: 2 in, 2 out]
            n182 = property on="Coeff_cl_ch3" class="Clust (strict)"("DisabledEnum"=w315) -> ()  [unwired: 2 in, 2 out]
            n183 = property on="Coeff_cl_ch4" class="Clust (strict)"("DisabledEnum"=w315) -> ()  [unwired: 2 in, 2 out]
            n184 = property on="Coeff_cl_ch5" class="Clust (strict)"("DisabledEnum"=w315) -> ()  [unwired: 2 in, 2 out]
            n185 = property on="Coeff_cl_ch6" class="Clust (strict)"("DisabledEnum"=w315) -> ()  [unwired: 2 in, 2 out]
            n186 = property on="Порт Блока 4" class="DigNum (strict)"("DisabledEnum"=w315) -> ()  [unwired: 2 in, 2 out]
            n187 = property on="IP Блока 3" class="Str"("DisabledEnum"=w315) -> ()  [unwired: 2 in, 2 out]
            n188 = property on="Coeff_cl_ch7" class="Clust (strict)"("DisabledEnum"=w315) -> ()  [unwired: 2 in, 2 out]
            n189 = property on="Порт Блока 3" class="DigNum (strict)"("DisabledEnum"=w315) -> ()  [unwired: 2 in, 2 out]
            n190 = property on="IP Блока 4" class="Str"("DisabledEnum"=w315) -> ()  [unwired: 2 in, 2 out]
            n191 = property on="Пароль" class="Str"("Value"="" ("Пароль")) -> ()  [unwired: 2 in, 2 out]
          }
        }
      }
      event "save_coeff.": Value Change {
        w318 = T4 0 items=["no dialog", "OK message", "continue or stop message", "OK message + warnings", "continue/stop + warnings"] ("type of dialog (OK msg:1)")
        n192 = event-data() -> ("OldVal"=w340:bool)  [unwired: 1 out]
        n193 = local write "save_coeff."(w340) -> ()
        n194 = property on="Coeff_cl_ch5" class="Clust (strict)"() -> (error out=w336:errorcluster, "Value"=w327:T1)  [unwired: 2 in, 1 out]
        n195 = property on="Coeff_cl_ch1" class="Clust (strict)"() -> (error out=w339:errorcluster, "Value"=w331:T1)  [unwired: 2 in, 1 out]
        n196 = property on="Coeff_cl_ch2" class="Clust (strict)"(error in=w339) -> (error out=w338:errorcluster, "Value"=w330:T1)  [unwired: 1 in, 1 out]
        n197 = property on="Coeff_cl_ch6" class="Clust (strict)"(error in=w336) -> (error out=w335:errorcluster, "Value"=w326:T1)  [unwired: 1 in, 1 out]
        n198 = property on="Coeff_cl_ch3" class="Clust (strict)"(error in=w338) -> (error out=w337:errorcluster, "Value"=w329:T1)  [unwired: 1 in, 1 out]
        n199 = property on="Coeff_cl_ch7" class="Clust (strict)"(error in=w335) -> (error out=w332:errorcluster, "Value"=w325:T1)  [unwired: 1 in, 1 out]
        n200 = property on="Coeff_cl_ch4" class="Clust (strict)"(error in=w337) -> (error out=w333:errorcluster, "Value"=w328:T1)  [unwired: 1 in, 1 out]
        n201 = call "Cluster_to_string_(SubVI).vi"("input cluster 1"=w327, "input cluster 2"=w326, "input cluster 3"=w325) -> ("string of coefficients"=w323:string, "error out"=w324:errorcluster)  [unwired: 11 in]
        n202 = Merge Errors(w333, w332, w324) -> (w334:errorcluster)
        n203 = call "Cluster_to_string_(SubVI).vi"("input cluster 1"=w331, "input cluster 2"=w330, "input cluster 3"=w329, "input cluster 4"=w328, "error in"=w334) -> ("string of coefficients"=w322:string, "error out"=w320:errorcluster)  [unwired: 9 in]
        n204 = Concatenate Strings(w322, w323) -> (w321:string)
        n205 = call "Create_and_save_to_file (SubVI).vi"("input string"=w321, "error in"=w320) -> ("Текущее расположение файла"=→"Путь к файлу с коэф.":path, "error out"=w319:errorcluster)  [unwired: 4 in]
        n206 = call <vilib>:"General Error Handler.vi"("type of dialog (OK msg:1)"=w318, "error in (no error)"=w319) -> ()  [unwired: 9 in, 5 out]
      }
      event "load_coeff.": Value Change {
        w343 = T4 0 items=["no dialog", "OK message", "continue or stop message", "OK message + warnings", "continue/stop + warnings"] ("type of dialog (OK msg:1)")
        n207 = event-data() -> ("OldVal"=w345:bool)  [unwired: 1 out]
        n208 = disable-structure shown="Enabled" {
          disable-tunnel: [w348 w351] -> w342
          disable-tunnel: [w347 w352] -> w344
          frame Disabled {
            n209 = Read from Text File(prompt (Open existing file)="Укажите  файл") -> (text=w347:string, cancelled=w349:bool, error out=w348:errorcluster)  [unwired: 3 in, 1 out]
          }
          frame Enabled {
            n210 = call <vilib>:"Application Directory.vi"() -> ("Application Directory"=w356:path)
            n211 = Path To String(path=w356) -> (string=w355:string)
            n212 = Concatenate Strings(w355, "\\Настройки.txt" ("prompt (Open existing file)")) -> (w354:string)
            n213 = String To Path(string=w354) -> (path=w350:path)
            n214 = local write "Путь к файлу с коэф."(w350) -> ()
            n215 = Read from Text File(file (use dialog)=w350) -> (text=w352:string, error out=w351:errorcluster)  [unwired: 3 in, 2 out]
          }
        }
        n216 = local write "load_coeff."(w345) -> ()
        n217 = case shown="No Error" w342 {
          selector: w342 -> [w360 w386]
          tunnel: w344 -> [w385 _]
          tunnel: [w357 w386] -> w341
          frame No Error {
            n218 = call "String_to_num (SubVI).vi"("String in"=w385, "error in"=w360) -> ("Rest of string OUT"=w382:string, "error out"=w383:errorcluster, "output cluster \nof coefficients"=w384:T8)  [unwired: 5 in]
            n219 = property on="Coeff_cl_ch1" class="Clust (strict)"(error in=w383, "Value"=w384) -> (error out=w381:errorcluster)  [unwired: 1 in, 1 out]
            n220 = call "String_to_num (SubVI).vi"("String in"=w382, "error in"=w381) -> ("Rest of string OUT"=w365:string, "error out"=w380:errorcluster, "output cluster \nof coefficients"=w379:T8)  [unwired: 5 in]
            n221 = property on="Coeff_cl_ch2" class="Clust (strict)"(error in=w380, "Value"=w379) -> (error out=w378:errorcluster)  [unwired: 1 in, 1 out]
            n222 = call "String_to_num (SubVI).vi"("String in"=w365, "error in"=w378) -> ("Rest of string OUT"=w366:string, "error out"=w377:errorcluster, "output cluster \nof coefficients"=w364:T8)  [unwired: 5 in]
            n223 = property on="Coeff_cl_ch3" class="Clust (strict)"(error in=w377, "Value"=w364) -> (error out=w376:errorcluster)  [unwired: 1 in, 1 out]
            n224 = call "String_to_num (SubVI).vi"("String in"=w366, "error in"=w376) -> ("Rest of string OUT"=w359:string, "error out"=w375:errorcluster, "output cluster \nof coefficients"=w363:T8)  [unwired: 5 in]
            n225 = property on="Coeff_cl_ch4" class="Clust (strict)"(error in=w375, "Value"=w363) -> (error out=w358:errorcluster)  [unwired: 1 in, 1 out]
            n226 = call "String_to_num (SubVI).vi"("String in"=w359, "error in"=w358) -> ("Rest of string OUT"=w367:string, "error out"=w374:errorcluster, "output cluster \nof coefficients"=w362:T8)  [unwired: 5 in]
            n227 = property on="Coeff_cl_ch5" class="Clust (strict)"(error in=w374, "Value"=w362) -> (error out=w373:errorcluster)  [unwired: 1 in, 1 out]
            n228 = call "String_to_num (SubVI).vi"("String in"=w367, "error in"=w373) -> ("Rest of string OUT"=w368:string, "error out"=w372:errorcluster, "output cluster \nof coefficients"=w361:T8)  [unwired: 5 in]
            n229 = property on="Coeff_cl_ch6" class="Clust (strict)"(error in=w372, "Value"=w361) -> (error out=w371:errorcluster)  [unwired: 1 in, 1 out]
            n230 = call "String_to_num (SubVI).vi"("String in"=w368, "error in"=w371) -> ("error out"=w370:errorcluster, "output cluster \nof coefficients"=w369:T8)  [unwired: 5 in, 1 out]
            n231 = property on="Coeff_cl_ch7" class="Clust (strict)"(error in=w370, "Value"=w369) -> (error out=w357:errorcluster)  [unwired: 1 in, 1 out]
          }
          frame Error {
            w387 = T1 {"k1"=0.0, "k2"=0.0, "k3"=0.0, "k4"=0.0, "k5"=0.0, "k6"=0.0, "k7"=0.0, "R0"=0.0} ("Coeff_cl_ch1")
            n232 = property on="Coeff_cl_ch1" class="Clust (strict)"("Value"=w387) -> ()  [unwired: 2 in, 2 out]
            n233 = property on="Coeff_cl_ch2" class="Clust (strict)"("Value"=w387) -> ()  [unwired: 2 in, 2 out]
            n234 = property on="Coeff_cl_ch3" class="Clust (strict)"("Value"=w387) -> ()  [unwired: 2 in, 2 out]
            n235 = property on="Coeff_cl_ch4" class="Clust (strict)"("Value"=w387) -> ()  [unwired: 2 in, 2 out]
            n236 = property on="Coeff_cl_ch5" class="Clust (strict)"("Value"=w387) -> ()  [unwired: 2 in, 2 out]
            n237 = property on="Coeff_cl_ch6" class="Clust (strict)"("Value"=w387) -> ()  [unwired: 2 in, 2 out]
            n238 = String To Path(string="Ошибка загрузки файла Настройки.txt") -> (path=w389:path)
            n239 = property on="Coeff_cl_ch7" class="Clust (strict)"("Value"=w387) -> ()  [unwired: 2 in, 2 out]
            n240 = local write "Путь к файлу с коэф."(w389) -> ()
          }
        }
        n241 = call <vilib>:"General Error Handler.vi"("type of dialog (OK msg:1)"=w343, "error in (no error)"=w341) -> ()  [unwired: 9 in, 5 out]
      }
      event Timeout {
        n242 = event-data() -> ()  [unwired: 2 out]
        n243 = local read "T1"() -> (w411:dbl)
        n244 = local read "T2"() -> (w410:dbl)
        n245 = local read "T3"() -> (w409:dbl)
        n246 = local read "T4"() -> (w406:dbl)
        n247 = local read "T5"() -> (w407:dbl)
        n248 = local read "T6"() -> (w408:dbl)
        n249 = local read "T7"() -> (w405:dbl)
        n250 = Merge Signals(w411) -> (w404:dynamicdata)
        n251 = Merge Signals(w410) -> (w403:dynamicdata)
        n252 = Merge Signals(w409) -> (w402:dynamicdata)
        n253 = Merge Signals(w406) -> (w401:dynamicdata)
        n254 = Merge Signals(w407) -> (w400:dynamicdata)
        n255 = Merge Signals(w408) -> (w399:dynamicdata)
        n256 = Merge Signals(w405) -> (w398:dynamicdata)
        n257 = Merge Signals(w404, w403, w402, w401, w400, w399, w398) -> (→"Graphs T":dynamicdata)
        n258 = local read "dT2"() -> (w395:dbl)
        n259 = local read "dT1"() -> (w396:dbl)
        n260 = local read "dT3"() -> (w394:dbl)
        n261 = Merge Signals(w396) -> (w392:dynamicdata)
        n262 = Merge Signals(w395) -> (w393:dynamicdata)
        n263 = Merge Signals(w394) -> (w391:dynamicdata)
        n264 = Merge Signals(w392, w393, w391) -> (→"Graphs dT":dynamicdata)
      }
      event "IP Блока 4", "Порт Блока 4", "IP Блока 3", "Порт Блока 3": Value Change {
        w424 = T4 0 items=["no dialog", "OK message", "continue or stop message", "OK message + warnings", "continue/stop + warnings"] ("type of dialog (OK msg:1)")
        # "сохр IP и порта в файл"
        n265 = event-data() -> ()  [unwired: 2 out]
        n266 = call <vilib>:"Application Directory.vi"() -> ("Application Directory"=w442:path)
        n267 = Path To String(path=w442) -> (string=w441:string)
        n268 = local read "IP Блока 4"() -> (w438:string)
        n269 = local read "Порт Блока 4"() -> (w437:u16)
        n270 = local read "IP Блока 3"() -> (w418:string)
        n271 = local read "Порт Блока 3"() -> (w419:u16)
        n272 = Concatenate Strings(w441, "\\IP.txt" ("prompt (Open existing file)")) -> (w440:string)
        n273 = String To Path(string=w440) -> (path=w425:path)
        n274 = Open/Create/Replace File(file path (use dialog)=w425, operation (0:open)=T7."replace or create") -> (refnum out=w428:refnum<file>, error out=w427:errorcluster)  [unwired: 1 in, 4 out]
        n275 = Number To Decimal String(number=w437) -> (decimal integer string=w433:string)  [unwired: 1 in]
        n276 = Number To Decimal String(number=w419) -> (decimal integer string=w420:string)  [unwired: 1 in]
        n277 = Concatenate Strings("%" ("string"), w438, "-" ("string")) -> (w434:string)
        n278 = Concatenate Strings("*" ("string"), w433, "--" ("string")) -> (w435:string)
        n279 = Concatenate Strings("%" ("string"), w418, "---" ("string")) -> (w417:string)
        n280 = Concatenate Strings("*" ("string"), w420, "----" ("string")) -> (w416:string)
        n281 = Concatenate Strings(w434, w435, w417, w416) -> (w436:string)
        n282 = Write to Text File(file (use dialog)=w428, text=w436, error in=w427) -> (refnum out=w430:refnum<file>, error out=w429:errorcluster)  [unwired: 2 out]
        n283 = Close File(refnum=w430, error in=w429) -> (error out=w423:errorcluster)  [unwired: 1 out]
        n284 = call <vilib>:"General Error Handler.vi"("type of dialog (OK msg:1)"=w424, "error in (no error)"=w423) -> ()  [unwired: 1 in, 13 out]
      }
    }
    n285 = Wait Until Next ms Multiple(millisecond multiple=u32 200) -> ()  [unwired: 1 out]
    n286 = local read "stop"() -> (w241:bool)
  }
  n287 = event shown="[0] \"stop\": Value Change" {
    selector: _ -> [_]
    dyn-events: _ -> [_]
    timeout: _ -> [_]
    event "stop": Value Change {
      w448 = T4 0 items=["no dialog", "OK message", "continue or stop message", "OK message + warnings", "continue/stop + warnings"] ("type of dialog (OK msg:1)")
      w446 = FALSE ("Запись в файл")
      n288 = event-data() -> ()  [unwired: 1 in, 1 out]
      n289 = local read "Блок 3"() -> (w451:refnum<class "Modbus Master.lvclass">)
      n290 = local read "Блок 4"() -> (w450:refnum<class "Modbus Master.lvclass">)
      n291 = property on="Запись в файл" class="Bool (strict)"("Value"=FALSE ("Запись в файл")) -> ()  [unwired: 2 in, 2 out]
      n292 = call-dynamic "Shutdown.vi"("Modbus master in"=w451) -> ("error out"=w452:errorcluster)  [unwired: 10 in]
      n293 = call-dynamic "Shutdown.vi"("Modbus master in"=w450) -> ("error out"=w449:errorcluster)  [unwired: 10 in]
      n294 = flat-sequence {
        tunnel: [w460] -> w444
        tunnel: w452 -> [w460]
        tunnel: w449 -> [w459]
        tunnel: [w459] -> w445
        frame #0 {
          n295 = Wait (ms)(milliseconds to wait=u32 100) -> ()  [unwired: 1 out]
        }
      }
      n296 = local read "refnum out"() -> (w455:refnum<file>)
      n297 = Merge Errors(w444, w445) -> (w443:errorcluster)
      n298 = Close File(refnum=w455, error in=w443) -> (error out=w454:errorcluster)  [unwired: 1 out]
      n299 = property on="Запись в файл" class="Bool (strict)"(error in=w454, "Value"=w446) -> (error out=w453:errorcluster)  [unwired: 1 in, 1 out]
      n300 = local write "Связь с блоком 4"(w446) -> ()
      n301 = flat-sequence {
        tunnel: w453 -> [w458]
        tunnel: [w458] -> w447
        frame #0 {
          n302 = Stop(stop? (T)=TRUE) -> ()
        }
      }
      n303 = local write "Связь с блоком 3"(w446) -> ()
      n304 = call <vilib>:"General Error Handler.vi"("error in (no error)"=w447, "[exception action] (none:0)"=w448) -> ()  [unwired: 2 in, 12 out]
    }
  }
  n305 = call <vilib>:"Application Directory.vi"() -> ("Application Directory"=w49:path)
  n306 = Path To String(path=w49) -> (string=w50:string)
  n307 = Concatenate Strings(w50, "\\IP.txt" ("prompt (Open existing file)")) -> (w51:string)
  n308 = String To Path(string=w51) -> (path=w53:path)
  n309 = local write "stop"(FALSE ("Boolean")) -> ()
  n310 = Read from Text File(file (use dialog)=w53) -> (refnum out=w37:refnum<file>, text=w55:string, error out=w42:errorcluster)  [unwired: 3 in, 1 out]
  n311 = property on="Graphs dT" class="WFChart (strict)"("YScale.ScaleFit"=u8 2 ("Y Scale.Scale Fit")) -> (error out=w13:errorcluster)  [unwired: 2 in, 1 out]
  n312 = property on="Graphs T" class="WFChart (strict)"("YScale.ScaleFit"=u8 2 ("Y Scale.Scale Fit")) -> (error out=w12:errorcluster)  [unwired: 2 in, 1 out]
  n313 = property on="мин." class="Str"("Disabled"=w72) -> (error out=w71:errorcluster)  [unwired: 2 in, 1 out]
  n314 = property on="Coeff_cl_ch1" class="Clust (strict)"("DisabledEnum"=w58) -> ()  [unwired: 2 in, 2 out]
  n315 = property on="Coeff_cl_ch2" class="Clust (strict)"("DisabledEnum"=w58) -> ()  [unwired: 2 in, 2 out]
  n316 = Match Pattern(string=w55, regular expression="*") -> (after substring=w29:string)  [unwired: 1 in, 3 out]
  n317 = Match Pattern(string=w55, regular expression="%") -> (after substring=w48:string)  [unwired: 1 in, 3 out]
  n318 = invoke on="Graphs dT" class="WFChart (strict)" method="Reinit To Default"(error in=w13) -> (error out=w64:errorcluster)  [unwired: 2 in, 2 out]
  n319 = invoke on="Graphs T" class="WFChart (strict)" method="Reinit To Default"(error in=w12) -> (error out=w8:errorcluster)  [unwired: 2 in, 2 out]
  n320 = property on="часы" class="Str"(error in=w71, "Disabled"=w72) -> (error out=w70:errorcluster)  [unwired: 1 in, 1 out]
  n321 = property on="Coeff_cl_ch3" class="Clust (strict)"("DisabledEnum"=w58) -> ()  [unwired: 2 in, 2 out]
  n322 = property on="Coeff_cl_ch4" class="Clust (strict)"("DisabledEnum"=w58) -> ()  [unwired: 2 in, 2 out]
  n323 = Match Pattern(string=w29, regular expression="--" ("string")) -> (before substring=w28:string, after substring=w20:string)  [unwired: 1 in, 2 out]
  n324 = Match Pattern(string=w20, regular expression="*") -> (after substring=w26:string)  [unwired: 1 in, 3 out]
  n325 = Match Pattern(string=w20, regular expression="%") -> (after substring=w25:string)  [unwired: 1 in, 3 out]
  n326 = Match Pattern(string=w26, regular expression="----" ("string")) -> (before substring=w27:string)  [unwired: 1 in, 3 out]
  n327 = Match Pattern(string=w25, regular expression="---" ("string")) -> (before substring=w45:string)  [unwired: 1 in, 3 out]
  n328 = invoke on="Добавить время" class="Ring (strict)" method="Reinit To Default"(error in=w70) -> (error out=w68:errorcluster)  [unwired: 2 in, 2 out]
  n329 = Match Pattern(string=w48, regular expression="-" ("string")) -> (before substring=w47:string)  [unwired: 1 in, 3 out]
  n330 = Scan From String(format string="%d", input string=w27, default 1=u16 0 ("default value 1")) -> (error out=w18:errorcluster, output 1=w44:u16)  [unwired: 2 in, 2 out]
  n331 = Scan From String(format string="%d", input string=w28, default 1=u16 0 ("default value 1")) -> (error out=w19:errorcluster, output 1=w46:u16)  [unwired: 2 in, 2 out]
  n332 = property on="Graphs dT" class="WFChart (strict)"(error in=w64, "Value"=dynamicdata [{"t0"=timestamp(3465273261.7246556 s since 1904-01-01), "dt"=1.0, "Y"=[0.1931097262457384]}, {"t0"=timestamp(3465273261.7246556 s since 1904-01-01), "dt"=1.0, "Y"=[0.3594116459482981]}, {"t0"=timestamp(3465273261.7246556 s since 1904-01-01), "dt"=1.0, "Y"=[0.8898205452798131]}, {"t0"=timestamp(3465273261.7246556 s since 1904-01-01), "dt"=1.0, "Y"=[0.747699236883661]}] ("Graphs")) -> (error out=w63:errorcluster)  [unwired: 1 in, 1 out]
  n333 = property on="Coeff_cl_ch5" class="Clust (strict)"("DisabledEnum"=w58) -> ()  [unwired: 2 in, 2 out]
  n334 = property on="Coeff_cl_ch6" class="Clust (strict)"("DisabledEnum"=w58) -> ()  [unwired: 2 in, 2 out]
  n335 = property on="Graphs T" class="WFChart (strict)"(error in=w8, "Value"=dynamicdata [{"t0"=timestamp(3465273261.7246556 s since 1904-01-01), "dt"=1.0, "Y"=[0.1931097262457384]}, {"t0"=timestamp(3465273261.7246556 s since 1904-01-01), "dt"=1.0, "Y"=[0.3594116459482981]}, {"t0"=timestamp(3465273261.7246556 s since 1904-01-01), "dt"=1.0, "Y"=[0.8898205452798131]}, {"t0"=timestamp(3465273261.7246556 s since 1904-01-01), "dt"=1.0, "Y"=[0.747699236883661]}] ("Graphs")) -> (error out=w9:errorcluster)  [unwired: 1 in, 1 out]
  n336 = Merge Errors(w19, w18, w42) -> (w43:errorcluster)
  n337 = invoke on="File header exist?" class="Bool (strict)" method="Reinit To Default"(error in=w68) -> (error out=w69:errorcluster)  [unwired: 2 in, 2 out]
  n338 = property on="Coeff_cl_ch7" class="Clust (strict)"("DisabledEnum"=w58) -> ()  [unwired: 2 in, 2 out]
  n339 = case shown="No Error" w43 {
    selector: w43 -> [w463 w468]
    tunnel: w47 -> [w467 _]
    tunnel: w46 -> [w466 _]
    tunnel: w45 -> [w465 _]
    tunnel: w44 -> [w464 _]
    tunnel: [w467 "?"] -> w41
    tunnel: [w466 u16 0 ("default value 1")] -> w40
    tunnel: [w465 "?"] -> w39
    tunnel: [w464 u16 0 ("default value 1")] -> w38
    tunnel: w37 -> [w462 w469]
    tunnel: [w462 w469] -> w36
    tunnel: [w463 w468] -> w35
    frame No Error {
    }
    frame Error {
    }
  }
  n340 = property on="Graphs dT" class="WFChart (strict)"(error in=w63, "History Data"=dynamicdata[] []) -> (error out=w67:errorcluster)  [unwired: 1 in, 1 out]
  n341 = property on="Graphs T" class="WFChart (strict)"(error in=w9, "History Data"=dynamicdata[] []) -> (error out=w6:errorcluster)  [unwired: 1 in, 1 out]
  n342 = property on="Расположение файла" class="Path"(error in=w69, "Disabled"=u8 2) -> ()  [unwired: 1 in, 2 out]
  n343 = local write "IP Блока 4"(w41) -> ()
  n344 = local write "IP Блока 3"(w39) -> ()
  n345 = local write "Порт Блока 4"(w40) -> ()
  n346 = local write "Порт Блока 3"(w38) -> ()
  n347 = property on="Graphs dT" class="WFChart (strict)"(error in=w67, "XScale.ScaleFit"=u8 0 ("Y Scale.Scale Fit")) -> ()  [unwired: 1 in, 2 out]
  n348 = property on="save_coeff." class="Bool (strict)"("DisabledEnum"=w58) -> ()  [unwired: 2 in, 2 out]
  n349 = property on="Graphs T" class="WFChart (strict)"(error in=w6, "XScale.ScaleFit"=u8 0 ("Y Scale.Scale Fit")) -> ()  [unwired: 1 in, 2 out]
  n350 = property on="load_coeff." class="Bool (strict)"("DisabledEnum"=w58) -> (error out=w56:errorcluster)  [unwired: 2 in, 1 out]
  n351 = disable-structure shown="Disabled" {
    frame Disabled {
      n352 = local read "File header exist?"() -> (w474:bool)
      n353 = case shown="True" w474 {
        tunnel: [w479 w502] -> _
        frame False {
          # "выполняется 1 раз"
          # "создание заголовка файла"
          n354 = call "Ch_data_title_pattern (SubVI).vi"("Единица измерений"="") -> ("error out"=w479:errorcluster, "Path"=→"Расположение файла":path, "Byte Stream File out"=→"refnum out":refnum<file>)  [unwired: 8 in]
          n355 = local write "File header exist?"(TRUE ("flag1")) -> ()
        }
        frame True {
          # "Сохранение результатов измерений и вывод на графики"
          n356 = local read "refnum out"() -> (w498:refnum<file>)
          n357 = local read "T2"() -> (w500:dbl)
          n358 = local read "T4"() -> (w486:dbl)
          n359 = local read "T3"() -> (w487:dbl)
          n360 = local read "T1"() -> (w501:dbl)
          n361 = local read item#-1() -> (w485)
          n362 = local read item#-1() -> (w482)
          n363 = Bundle("T1"=w501, "T2"=w500, "T3"=w487, "T4"=w486, w485, w482) -> (w499:T9)  [unwired: 1 in]
          n364 = call "Ch_data_pattern_8_save (SubVI).vi"("T Cluster"=w499, "file"=w498) -> ("error out"=w502:errorcluster)  [unwired: 25 in]
          n365 = Refnum to Path(1:w498) -> (0:w497:path)
          n366 = Unbundle(w499) -> ("T1"=w491:dbl, "T2"=w490:dbl, "T3"=w489:dbl, "T4"=w488:dbl, w483, w480)
          n367 = Path To String(path=w497) -> (string=→"Path":string)
          n368 = Merge Signals(w491) -> (w493:dynamicdata)
          n369 = Merge Signals(w490) -> (w494:dynamicdata)
          n370 = Merge Signals(w489) -> (w495:dynamicdata)
          n371 = Merge Signals(w488) -> (w492:dynamicdata)
          n372 = Merge Signals(w483) -> (w484:dynamicdata)
          n373 = Merge Signals(w480) -> (w481:dynamicdata)
          n374 = Merge Signals(w493, w494, w495, w492, w484, w481) -> ()  [unwired: 1 out]
        }
      }
    }
    frame Enabled {
    }
  }
  n375 = Close File(refnum=w36, error in=w35) -> (error out=w34:errorcluster)  [unwired: 1 out]
  n376 = property on="load_coeff." class="Bool (strict)"(error in=w56, "Val(Sgnl)"=TRUE ("Value (Signaling)")) -> ()  [unwired: 1 in, 2 out]
  n377 = property on="Graphs T" class="WFChart (strict)"() -> (error out=w3:errorcluster, "XScale.Minimum"=w4:dbl)  [unwired: 2 in, 1 out]
  n378 = property on="Graphs T" class="WFChart (strict)"() -> (error out=w1:errorcluster, "XScale.Maximum"=w2:dbl)  [unwired: 2 in, 1 out]
  n379 = call <vilib>:"General Error Handler.vi"("type of dialog (OK msg:1)"=w14, "error in (no error)"=w34) -> ()  [unwired: 1 in, 13 out]
  n380 = property on="Graphs dT" class="WFChart (strict)"(error in=w1, "XScale.Maximum"=w2) -> ()  [unwired: 1 in, 2 out]
  n381 = property on="Graphs dT" class="WFChart (strict)"(error in=w3, "XScale.Minimum"=w4) -> ()  [unwired: 1 in, 2 out]
  "File header exist?" <- FALSE ("flag1")
